vi "11.2.5.-Momentos Invariantes de Hu - h1, h2, h3, ..., h7.vi"(0 "n12":dbl, 1 "n11":dbl, 5 "n02":dbl, 7 "n20":dbl, 9 "n21":dbl, 11 "n03":dbl, 12 "n30":dbl) -> (8 "Momentos de Hu":dbl[](array[numeric]))   [LabVIEW 2020]
panel:
  # "Visión Artificial - Momentos Invariantes de Hu\nDiego Cervantes Rodríguez\ndicer0.com"
  # "h1 = n20+n02\nh2 = ((n20-n02)^2)+((2*n11)^2)\nh3 = ((n30-3*n12)^2)+((3*n21-n03)^2)\nh4 = ((n30+n12)^2)+((n21+n03)^2)\nh5 = ((n30-3*n12)*(n30+n12)*((n30+n12)^2 -3*(n21+n03)^2))+((3*n21-n03)*(n21+n03)*(3*(n30+n12)^2 -(n21+n03)^2))\nh6 = ((n20-n02)*((n30+n12)^2 -(n21+n03)^2)))+((4*n11)*(n30+n12)*(n21+n03))\nh7 = ((3*n21-n03)*(n30+n12)*((n30+n12)^2 -3*(n21+n03)^2))+((n30-3*n12)*(n21+n03)*(3*(n30+n12)^2 -(n21+n03)^2))"
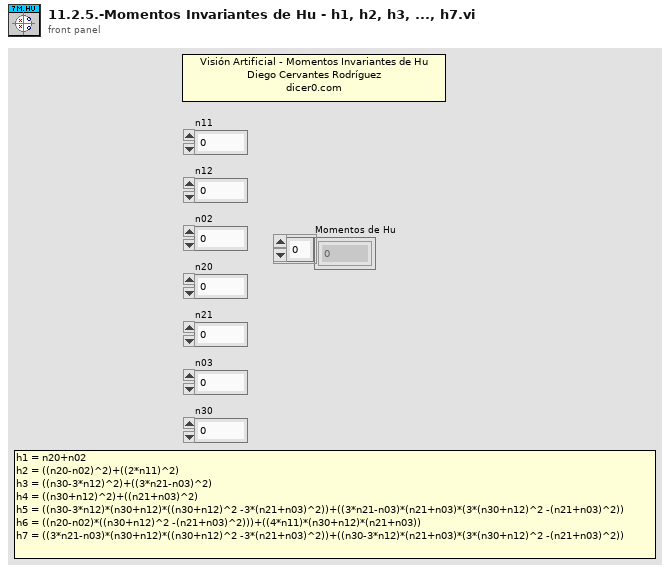
[diagram p1: front panel]
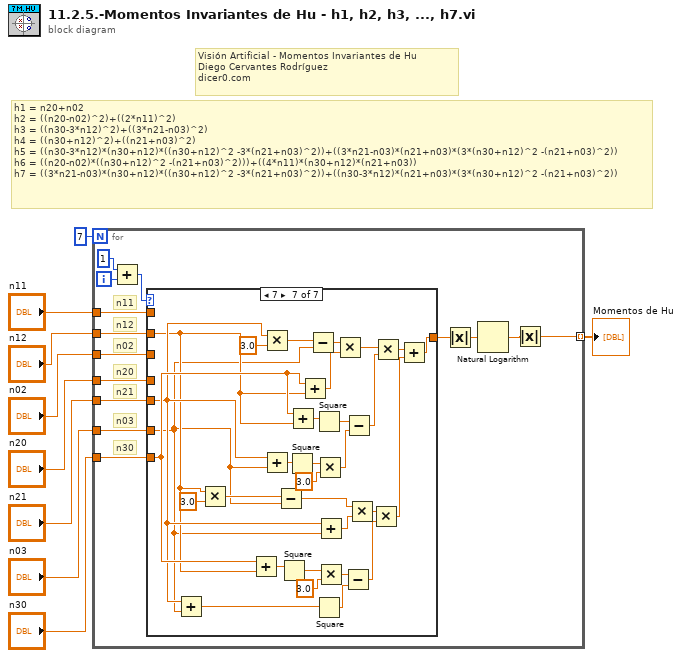
[diagram p0: block diagram]
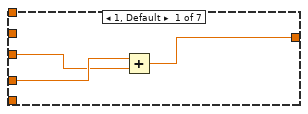
[diagram p2: hidden frame]
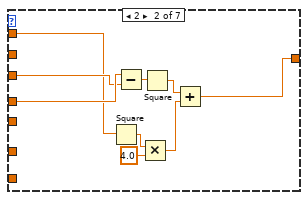
[diagram p3: hidden frame]
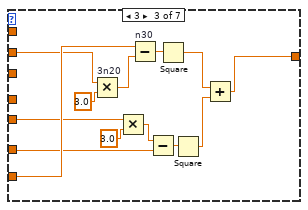
[diagram p4: hidden frame]
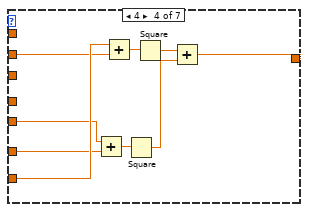
[diagram p5: hidden frame]
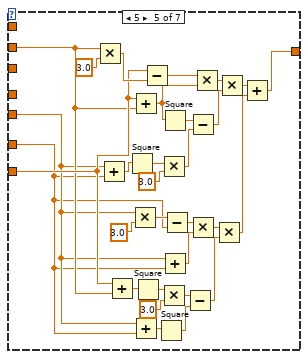
[diagram p6: hidden frame]
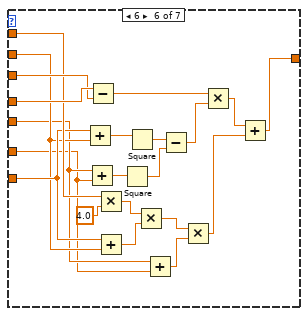
[diagram p7: hidden frame]
diagram:
  # "h1 = n20+n02\nh2 = ((n20-n02)^2)+((2*n11)^2)\nh3 = ((n30-3*n12)^2)+((3*n21-n03)^2)\nh4 = ((n30+n12)^2)+((n21+n03)^2)\nh5 = ((n30-3*n12)*(n30+n12)*((n30+n12)^2 -3*(n21+n03)^2))+((3*n21-n03)*(n21+n03)*(3*(n30+n12)^2 -(n21+n03)^2))\nh6 = ((n20-n02)*((n30+n12)^2 -(n21+n03)^2)))+((4*n11)*(n30+n12)*(n21+n03))\nh7 = ((3*n21-n03)*(n30+n12)*((n30+n12)^2 -3*(n21+n03)^2))+((n30-3*n12)*(n21+n03)*(3*(n30+n12)^2 -(n21+n03)^2))"
  # "Visión Artificial - Momentos Invariantes de Hu\nDiego Cervantes Rodríguez\ndicer0.com"
  n1 = for {
    N: 7 -> [_]
    tunnel: [w12] -> w8 mode=indexing
    tunnel: "n11" -> [w23]
    tunnel: "n12" -> [w22]
    tunnel: "n02" -> [w21]
    tunnel: "n20" -> [w20]
    tunnel: "n21" -> [w19]
    tunnel: "n03" -> [w18]
    tunnel: "n30" -> [w17]
    i -> [w16]
    # "n30"
    # "n03"
    # "n21"
    # "n20"
    # "n02"
    # "n12"
    # "n11"
    n2 = Add(x=1, y=w16) -> (x+y=w15:i32)
    n3 = case shown="7" w15 {
      tunnel: [w24 w30 w36 w49 w58 w88 w109] -> w13
      tunnel: w23 -> [_ w29 _ _ _ w93 _]
      tunnel: w22 -> [_ _ w39 w52 w61 w91 w113]
      tunnel: w21 -> [w25 w31 _ _ _ w95 _]
      tunnel: w20 -> [w26 w32 _ _ _ w96 _]
      tunnel: w19 -> [_ _ w38 w51 w60 w90 w114]
      tunnel: w18 -> [_ _ w37 w50 w59 w89 w112]
      tunnel: w17 -> [_ _ w40 w53 w62 w92 w115]
      frame 1, Default {
        n4 = Add(x=w26, y=w25) -> (x+y=w24:dbl)
      }
      frame 2 {
        n5 = Square(x=w29) -> (x^2=w28:dbl)
        n6 = Subtract(x=w32, y=w31) -> (x-y=w33:dbl)
        n7 = Multiply(x=w28, y=4.0) -> (x*y=w27:dbl)
        n8 = Square(x=w33) -> (x^2=w34:dbl)
        n9 = Add(x=w34, y=w27) -> (x+y=w30:dbl)
      }
      frame 3 {
        n10 = Multiply "3n20"(x=w39, y=3.0) -> (x*y=w46:dbl)
        n11 = Multiply(x=w38, y=3.0) -> (x*y=w43:dbl)
        n12 = Subtract "n30"(x=w40, y=w46) -> (x-y=w45:dbl)
        n13 = Subtract(x=w43, y=w37) -> (x-y=w42:dbl)
        n14 = Square(x=w45) -> (x^2=w44:dbl)
        n15 = Square(x=w42) -> (x^2=w41:dbl)
        n16 = Add(x=w44, y=w41) -> (x+y=w36:dbl)
      }
      frame 4 {
        n17 = Add(x=w51, y=w50) -> (x+y=w56:dbl)
        n18 = Add(x=w53, y=w52) -> (x+y=w57:dbl)
        n19 = Square(x=w56) -> (x^2=w54:dbl)
        n20 = Square(x=w57) -> (x^2=w55:dbl)
        n21 = Add(x=w55, y=w54) -> (x+y=w49:dbl)
      }
      frame 5 {
        n22 = Multiply(x=w61, y=3.0) -> (x*y=w64:dbl)
        n23 = Add(x=w60, y=w59) -> (x+y=w84:dbl)
        n24 = Add(x=w62, y=w61) -> (x+y=w72:dbl)
        n25 = Square(x=w84) -> (x^2=w83:dbl)
        n26 = Multiply(x=w60, y=3.0) -> (x*y=w77:dbl)
        n27 = Add(x=w62, y=w61) -> (x+y=w63:dbl)
        n28 = Add(x=w60, y=w59) -> (x+y=w68:dbl)
        n29 = Square(x=w72) -> (x^2=w71:dbl)
        n30 = Subtract(x=w62, y=w64) -> (x-y=w87:dbl)
        n31 = Square(x=w68) -> (x^2=w67:dbl)
        n32 = Multiply(x=w83, y=3.0) -> (x*y=w81:dbl)
        n33 = Multiply(x=w71, y=3.0) -> (x*y=w69:dbl)
        n34 = Square(x=w63) -> (x^2=w85:dbl)
        n35 = Add(x=w60, y=w59) -> (x+y=w75:dbl)
        n36 = Subtract(x=w77, y=w59) -> (x-y=w76:dbl)
        n37 = Subtract(x=w69, y=w67) -> (x-y=w66:dbl)
        n38 = Subtract(x=w85, y=w81) -> (x-y=w80:dbl)
        n39 = Multiply(x=w76, y=w75) -> (x*y=w74:dbl)
        n40 = Multiply(x=w87, y=w63) -> (x*y=w86:dbl)
        n41 = Multiply(x=w74, y=w66) -> (x*y=w73:dbl)
        n42 = Multiply(x=w86, y=w80) -> (x*y=w79:dbl)
        n43 = Add(x=w79, y=w73) -> (x+y=w58:dbl)
      }
      frame 6 {
        n44 = Add(x=w92, y=w91) -> (x+y=w107:dbl)
        n45 = Add(x=w90, y=w89) -> (x+y=w105:dbl)
        n46 = Subtract(x=w96, y=w95) -> (x-y=w108:dbl)
        n47 = Multiply(x=w93, y=4.0) -> (x*y=w101:dbl)
        n48 = Add(x=w92, y=w91) -> (x+y=w100:dbl)
        n49 = Square(x=w105) -> (x^2=w104:dbl)
        n50 = Square(x=w107) -> (x^2=w106:dbl)
        n51 = Multiply(x=w101, y=w100) -> (x*y=w99:dbl)
        n52 = Add(x=w90, y=w89) -> (x+y=w98:dbl)
        n53 = Subtract(x=w106, y=w104) -> (x-y=w94:dbl)
        n54 = Multiply(x=w99, y=w98) -> (x*y=w97:dbl)
        n55 = Multiply(x=w108, y=w94) -> (x*y=w103:dbl)
        n56 = Add(x=w103, y=w97) -> (x+y=w88:dbl)
      }
      frame 7 {
        n57 = Add(x=w114, y=w112) -> (x+y=w124:dbl)
        n58 = Multiply(x=w113, y=3.0) -> (x*y=w129:dbl)
        n59 = Add(x=w115, y=w113) -> (x+y=w125:dbl)
        n60 = Multiply(x=w114, y=3.0) -> (x*y=w138:dbl)
        n61 = Add(x=w114, y=w112) -> (x+y=w132:dbl)
        n62 = Subtract(x=w129, y=w112) -> (x-y=w128:dbl)
        n63 = Square(x=w125) -> (x^2=w120:dbl)
        n64 = Square(x=w132) -> (x^2=w117:dbl)
        n65 = Add(x=w115, y=w113) -> (x+y=w134:dbl)
        n66 = Add(x=w115, y=w113) -> (x+y=w136:dbl)
        n67 = Subtract(x=w138, y=w112) -> (x-y=w137:dbl)
        n68 = Square(x=w134) -> (x^2=w133:dbl)
        n69 = Square(x=w124) -> (x^2=w111:dbl)
        n70 = Multiply(x=w117, y=3.0) -> (x*y=w116:dbl)
        n71 = Add(x=w114, y=w112) -> (x+y=w127:dbl)
        n72 = Multiply(x=w120, y=3.0) -> (x*y=w119:dbl)
        n73 = Multiply(x=w137, y=w136) -> (x*y=w135:dbl)
        n74 = Subtract(x=w119, y=w111) -> (x-y=w123:dbl)
        n75 = Subtract(x=w133, y=w116) -> (x-y=w131:dbl)
        n76 = Multiply(x=w128, y=w127) -> (x*y=w126:dbl)
        n77 = Multiply(x=w126, y=w123) -> (x*y=w122:dbl)
        n78 = Multiply(x=w135, y=w131) -> (x*y=w110:dbl)
        n79 = Add(x=w110, y=w122) -> (x+y=w109:dbl)
      }
    }
    n80 = Absolute Value(x=w13) -> (abs(x)=w10:dbl)
    n81 = Natural Logarithm(1:w10) -> (0:w11:dbl)
    n82 = Absolute Value(x=w11) -> (abs(x)=w12:dbl)
  }
  "Momentos de Hu" <- w8
